vi "出力フォルダを作成する.vi"(8 "error in (no error)":errorcluster caption="エラー入力（エラーなし）", 9 "時刻":timestamp, 10 "現在時刻のサブフォルダを作成する?(F)":bool, 11 "ルートフォルダ":path) -> (0 "error out":errorcluster caption="エラー出力", 1 "ファイル名(拡張子なし)":string, 2 "ファイル名":string, 3 "作成されたパス":path)   [LabVIEW 2018]
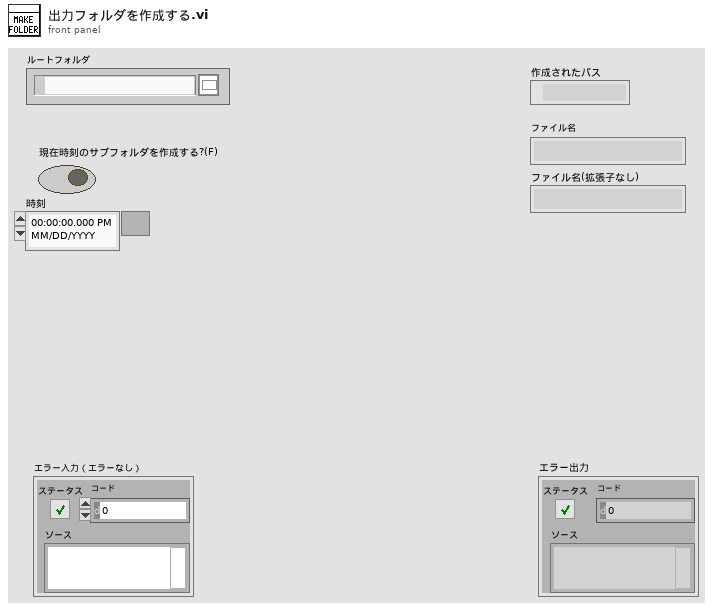
[diagram p1: front panel]
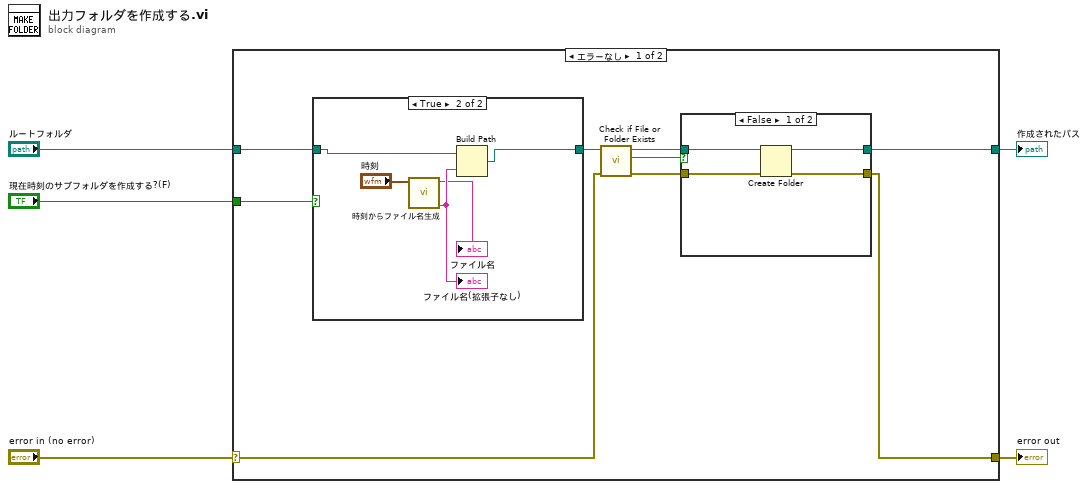
[diagram p0: block diagram]
diagram:
  n1 = case shown="エラーなし" "error in (no error)" {
    selector: "error in (no error)" -> [w7 w27]
    tunnel: [w11 w27] -> w4
    tunnel: "ルートフォルダ" -> [w9 _]
    tunnel: "現在時刻のサブフォルダを作成する?(F)" -> [w10 _]
    tunnel: [w6 _] -> w1
    frame No Error {
      n2 = case shown="TRUE" w10 {
        tunnel: w9 -> [w15 w20]
        tunnel: [w15 w18] -> w8
        frame False {
        }
        frame True {
          n3 = call "時刻からファイル名生成.vi"("時刻"="時刻") -> ("ファイル名(拡張子なし)"=w19:string, "ファイル名"=→"ファイル名":string)  [unwired: 9 in]
          "ファイル名(拡張子なし)" <- w19
          n4 = Build Path(base path=w20, name or relative path=w19) -> (appended path=w18:path)
        }
      }
      n5 = call <vilib>:"Check if File or Folder Exists.vi"("error in (no error)"=w7, "path"=w8) -> ("error out"=w12:errorcluster, "file or folder exists?"=w14:bool, "dup path"=w13:path)  [unwired: 7 in]
      n6 = case shown="FALSE" w14 {
        tunnel: w13 -> [w24 w26]
        tunnel: w12 -> [w23 w25]
        tunnel: [w22 w26] -> w6
        tunnel: [w21 w25] -> w11
        frame False {
          n7 = Create Folder(path (use dialog)=w24, error in=w23) -> (created path=w22:path, error out=w21:errorcluster)  [unwired: 1 in, 1 out]
        }
        frame True {
        }
      }
    }
    frame Error {
    }
  }
  "error out" <- w4
  "作成されたパス" <- w1
